vi "pUSH_QUERY.vi"(10 "columns":string[](array[string]), 11 "Table Name":string) -> (3 "resulting string":string)   [LabVIEW 2020]
uses:
  <vilib>/regexp/Match Regular Expression.xnode
panel:
  out "whole match":string
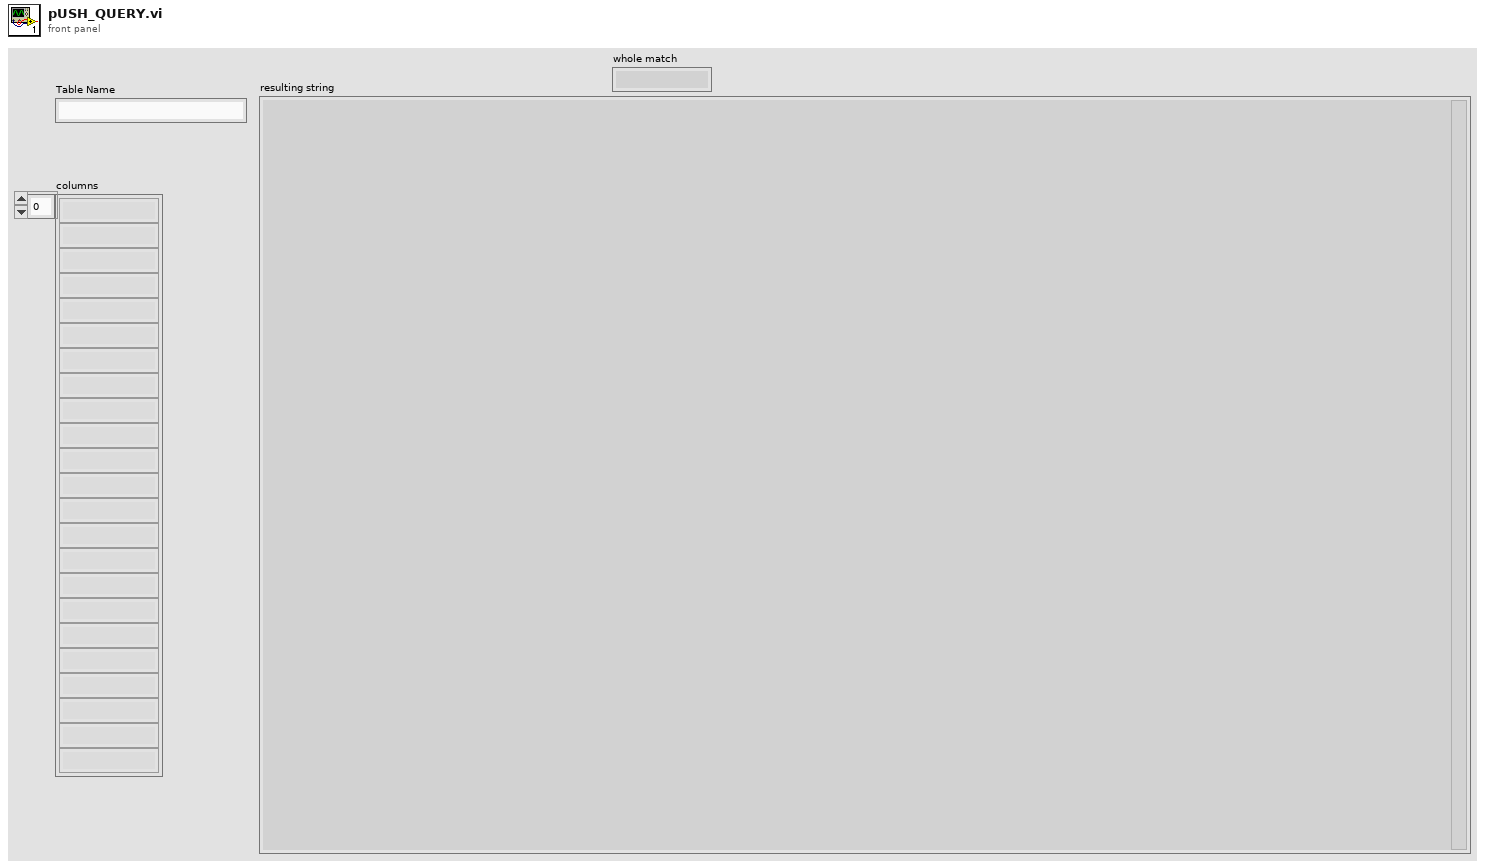
[diagram p1: front panel]
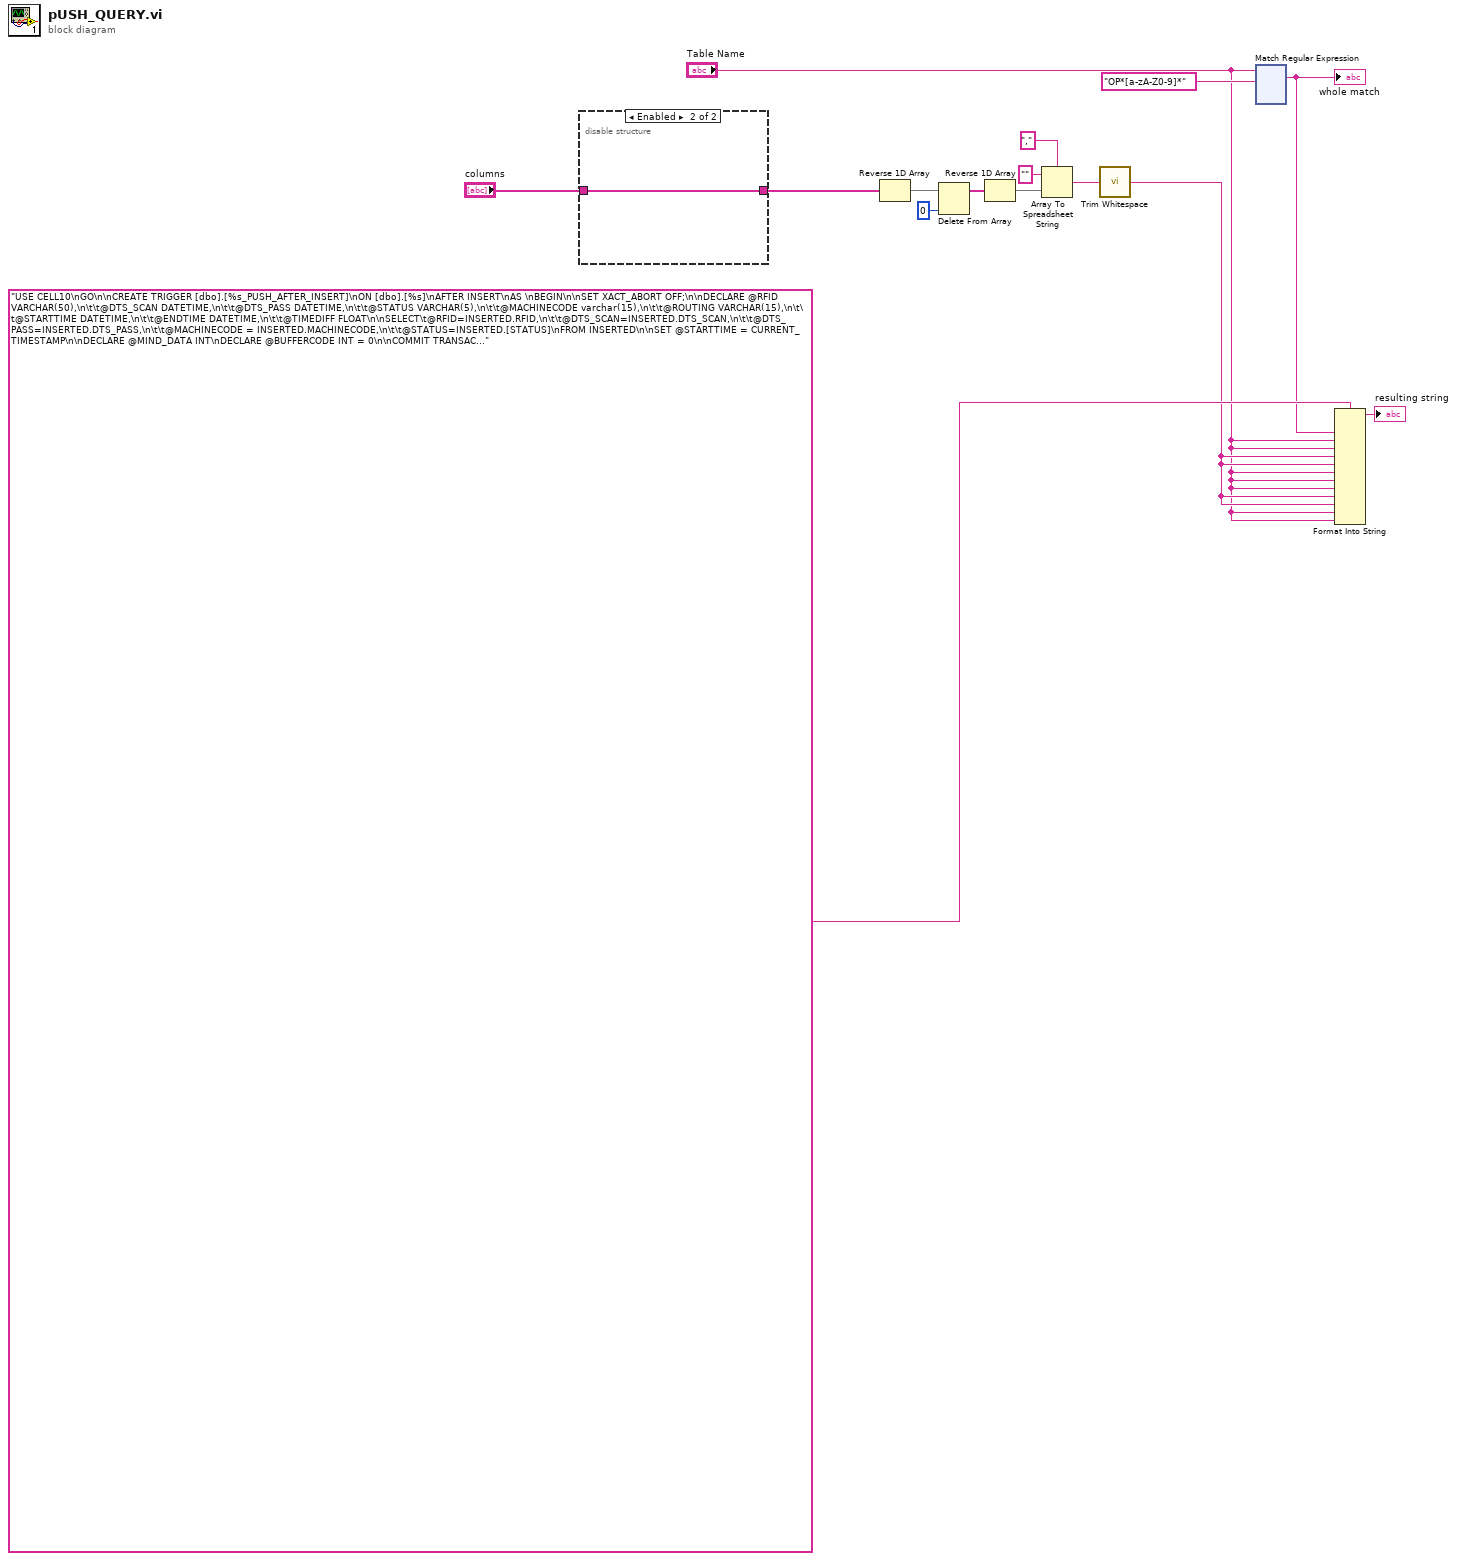
[diagram p0: block diagram]
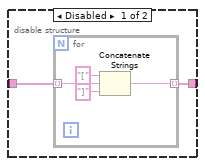
[diagram p2: hidden frame]
diagram:
  n1 = disable-structure shown="Enabled" {
    disable-tunnel: "columns" -> [w17 w22]
    disable-tunnel: [w16 w22] -> w4
    frame Disabled {
      n2 = for {
        tunnel: w17 -> [w21] mode=indexing
        tunnel: [w18] -> w16 mode=indexing
        n3 = Concatenate Strings("[" ("string"), w21, "]" ("string")) -> (w18:string)
      }
    }
    frame Enabled {
    }
  }
  n4 = Reverse 1D Array(array=w4) -> (reversed array=w11:string[])
  n5 = Delete From Array(array=w11, index=0) -> (array with subset deleted=w9:string[])  [unwired: 1 in, 1 out]
  n6 = Reverse 1D Array(array=w9) -> (reversed array=w8:string[])
  n7 = Array To Spreadsheet String(delimiter (Tab)=",", array=w8, 3:"" ("format string")) -> (spreadsheet string=w3:string)
  n8 = call <vilib>:"Trim Whitespace.vi"("string"=w3) -> ("trimmed string"=w2:string)  [unwired: 1 in]
  n9 = xnode "Match Regular Expression"("input string"="Table Name", "regular expression"="OP*[a-zA-Z0-9]*" ("String")) -> ("whole match"=w13:string)  [unwired: 4 in, 4 out]
  "whole match" <- w13
  n10 = Format Into String(format string="USE CELL10\nGO\n\nCREATE TRIGGER [dbo].[%s_PUSH_AFTER_INSERT]\nON [dbo].[%s]\nAFTER INSERT\nAS \nBEGIN\n\nSET XACT_ABORT OFF;\n\nDECLARE @RFID VARCHAR(50),\n\t\t@DTS_SCAN DATETIME,\n\t\t@DTS_PASS DATETIME,\n\t\t@STATUS VARCHAR(5),\n\t\t@MACHINECODE varchar(15),\n\t\t@ROUTING VARCHAR(15),\n\t\t@STARTTIME DATETIME,\n\t\t@ENDTIME DATETIME,\n\t\t@TIMEDIFF FLOAT\n\nSELECT\t@RFID=INSERTED.RFID,\n\t\t@DTS_SCAN=INSERTED.DTS_SCAN,\n\t\t@DTS_PASS=INSERTED.DTS_PASS,\n\t\t@MACHINECODE = INSERTED.MACHINECODE,\n\t\t@STATUS=INSERTED.[STATUS]\nFROM INSERTED\n\nSET @STARTTIME = CURRENT_TIMESTAMP\n\nDECLARE @MIND_DATA INT\nDECLARE @BUFFERCODE INT = 0\n\nCOMMIT TRANSACTION\n\nSELECT @MIND_DATA = [Mind_Data] FROM [dbo].[TD_SYSTEM_INFO] WHERE [STS_CD] = 0\nPRINT 'MIND'\nPRINT @MIND_DATA\nIF @MIND_DATA = 1\nSET @BUFFERCODE = 1\n\nBEGIN \n\nBEGIN TRY\nDECLARE @CMD1 NVARCHAR(MAX);\nDECLARE @CMD2 NVARCHAR(MAX);\n--PRINT 'MIND DEV'\nSET @CMD1 = 'INSERT INTO [MIND_LINK_SERVER].[BTS_CELL10].[DBO].[%s] \n\t\t\t\t(%s)\n\t\t(SELECT  %s FROM [dbo].[%s] WHERE RFID='+''''+ @RFID+''''+' AND DTS_PASS = '+''''+ @DTS_PASS+''''+' )'\n\nEXEC SP_EXECUTESQL @CMD1;\n\nEND TRY\t\nBEGIN CATCH\n--PRINT 'MIND BUFFER'\nSET @BUFFERCODE = 21603\nINSERT INTO [dbo].[TD_MIND_BUFFER] VALUES(@RFID,'',@MACHINECODE,@DTS_PASS,CURRENT_TIMESTAMP,0)\nEND CATCH\n\nUPDATE [dbo].[%s] SET [TS_FLAG] = @BUFFERCODE WHERE RFID = @RFID AND @DTS_SCAN = @DTS_SCAN\n\nEND\n\nIF @BUFFERCODE = 1 and @MIND_DATA = 1\nBEGIN\nSET @CMD1 = 'INSERT INTO [MIND_LINK_SERVER].[BTS_CELL10].[DBO].[%s] \n\t\t\t\t(%s)\n\t\t(SELECT %s FROM [dbo].[%s] WHERE [TS_FLAG] = 21603)'\n\nEXEC SP_EXECUTESQL @CMD1;\n\nUPDATE [dbo].[%s] SET [TS_FLAG] = 2 WHERE [TS_FLAG] = 21603\nEND\n\nBEGIN TRANSACTION\n\nSET @ENDTIME = CURRENT_TIMESTAMP\n\nSET @TIMEDIFF = DATEDIFF(MILLISECOND,@STARTTIME,@ENDTIME)\n\nINSERT INTO TD_TIME_LOG (RFID,Machinecode,Runtime,TGTRuntime,RunDate) values(@RFID,@MACHINECODE,@TIMEDIFF,'0',CURRENT_TIMESTAMP)\n\nEND" ("Table Name"), w13, "Table Name", "Table Name", w2, w2, "Table Name", "Table Name", "Table Name", w2, w2, "Table Name", "Table Name") -> (resulting string=→"resulting string":string)  [unwired: 2 in, 1 out]
